vi "Read Power.vi"(8 "error in":errorcluster, 11 "LTB-1 in":refnum<class "LTB-1.lvclass">) -> (0 "error out":errorcluster, 2 "Power (uW)":dbl, 3 "LTB-1 out":refnum<class "LTB-1.lvclass">, 4 "Power dBm":dbl)   [LabVIEW 2018, in "LTB-1.lvlib" / "LTB-1.lvclass"]
doc: "This is a dynamically dispatched VI. The child class will return the power levels in microWatts measured by the variable optical attenuator. VOA Power meter reports in dB - use appropriate equations to convert from dB to uW.\n\nAuthor: Ron Dexter\nCompany: Luminar\nModified: 5/20/2018"
uses:
  LTB-1.lvclass
  C:/AME Test Engineering/LabVIEW/PPLs/EXFO/Parent/EXFO.lvlibp/EXFO.lvclass
  LTB-1.lvclass/LTB-1.ctl
  PPLs/EXFO/Parent/EXFO.lvlibp/Methods/Read Resource.vi
  3150 Driver/3150.lvlib
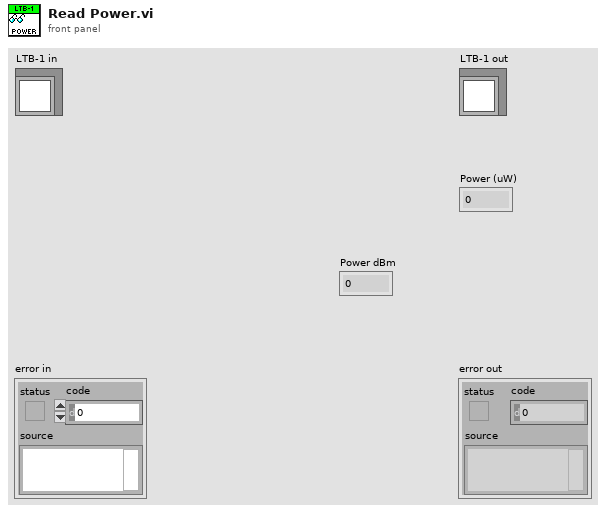
[diagram p1: front panel]
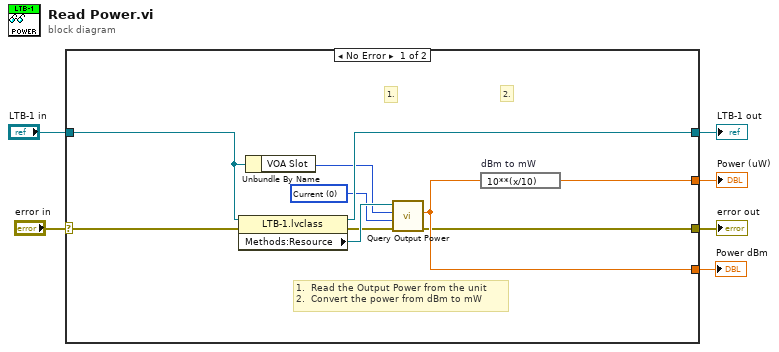
[diagram p0: block diagram]
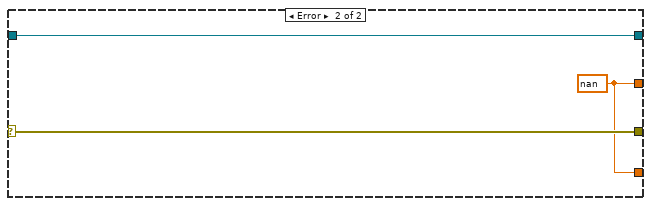
[diagram p2: hidden frame]
diagram:
  n1 = case shown="No Error" "error in" {
    selector: "error in" -> [w14 w18]
    tunnel: "LTB-1 in" -> [w13 w19]
    tunnel: [w16 w19] -> w5
    tunnel: [w15 w17] -> w4
    tunnel: [w7 w18] -> w3
    tunnel: [w8 w17] -> w1
    frame No Error {
      w10 = u16 0 items=["Current", "MINimum", "MAXimum", "DEFault"] ("Output Power Type (0:Current)")
      # "1.  Read the Output Power from the unit\n2.  Convert the power from dBm to mW"
      # "2."
      # "1."
      n2 = property class="LTB-1.lvclass"(reference=w13, error in=w14) -> (reference out=w16:refnum<class "LTB-1.lvclass">, error out=w11:errorcluster, "Methods:Resource"=w12:refnum<visa-resource-name>)
      n3 = Unbundle By Name(w13) -> ("VOA Slot"=w9:i16)
      n4 = call "Query Output Power.vi"("error in (no error)"=w11, "Output Power Type (0:Current)"=w10, "Platform Slot Number (10)"=w9, "VISA resource name"=w12) -> ("error out"=w7:errorcluster, "Output Power"=w8:dbl)  [unwired: 5 in, 1 out]
      n5 = expression code="10**(x/10)" "dBm to mW"(w8) -> (w15:dbl)
    }
    frame Error {
      w17 = nan ("Output Power")
    }
  }
  "error out" <- w3
  "LTB-1 out" <- w5
  "Power (uW)" <- w4
  "Power dBm" <- w1
